vi "ReadTrialList.vi"(11 "InputList":path) -> (2 "TrialList":T1[](array[typedef]))   [LabVIEW 2018]
uses:
  TrialListElements.ctl
  trial type.ctl
  rewtype.ctl
  <vilib>/Utility/file.llb/Read Delimited Spreadsheet (DBL).vi
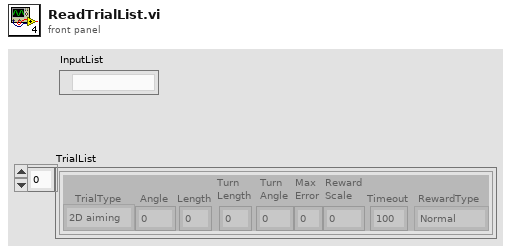
[diagram p1: front panel]
types:
  T1 = typedef "TrialListElements.ctl" = cluster{"TrialType":T2, "Angle":dbl, "Length":dbl, "TurnLength":dbl, "TurnAngle":dbl, "MaxError":dbl, "RewardScale":dbl, "Timeout":i32, "RewardType":T3}
  T2 = typedef "trial type.ctl" = enum8{"Linear", "2D aiming", "Two-part"}
  T3 = typedef "rewtype.ctl" = enum16{"Normal", "No reward"}
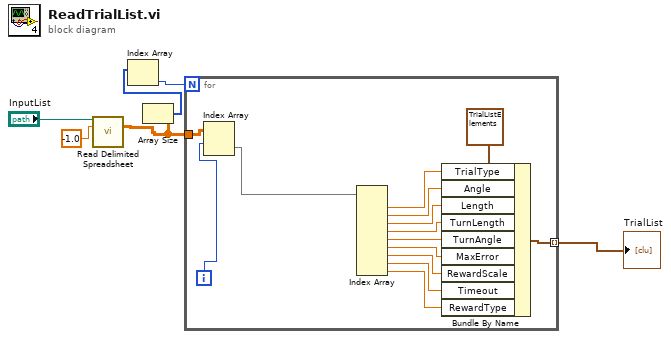
[diagram p0: block diagram]
diagram:
  n1 = call-poly <vilib>:"Read Delimited Spreadsheet.vi"("file path (dialog if empty)"="InputList", "number of rows (all:-1)"=-1.0) -> ("all rows"=w1:dbl[][])  [unwired: 8 in, 5 out]
  n2 = Array Size(array=w1) -> (size(s)=w3:i32[])
  n3 = Index Array(array=w3) -> (element=w2:i32)  [unwired: 1 in]
  n4 = for {
    N: w2 -> [_]
    tunnel: [w19] -> w4 mode=indexing
    tunnel: w1 -> [w18]
    i -> [w16]
    n5 = Index Array(array=w18, index (row)=w16) -> (element=w17:dbl[])  [unwired: 1 in]
    n6 = Index Array(array=w17) -> (element #1=w15:dbl, element #2=w14:dbl, element #3=w13:dbl, element #4=w12:dbl, element #5=w11:dbl, element #6=w10:dbl, element #7=w9:dbl, element #8=w8:dbl, element #9=w7:dbl)  [unwired: 9 in]
    n7 = Bundle By Name(cluster=T1 {"TrialType"=enum."2D aiming", "Angle"=0.0, "Length"=0.0, "TurnLength"=0.0, "TurnAngle"=0.0, "MaxError"=0.0, "RewardScale"=0.0, "Timeout"=100, "RewardType"=enum."Normal"} ("TrialListElements"), "TrialType"=w15, "Angle"=w14, "Length"=w13, "TurnLength"=w12, "TurnAngle"=w11, "MaxError"=w10, "RewardScale"=w9, "Timeout"=w8, "RewardType"=w7) -> (w19:T1)
  }
  "TrialList" <- w4
